vi "Generate Web Service Privilege.vi"(8 "error in (no error)":errorcluster, 10 "Service Name":string, 11 "data.Privilege Mapping":T1(array[cluster])) -> (0 "error out":errorcluster, 3 "resulting string":string)   [LabVIEW 2020, in "Web Service Description.lvlib"]
uses:
  <vilib>/AppBuilder/Engine/WebServiceDescription/Web Service Description.lvlib
  <vilib>/AppBuilder/Engine/WebServiceDescription/XMLGen/XMLGen.lvlib
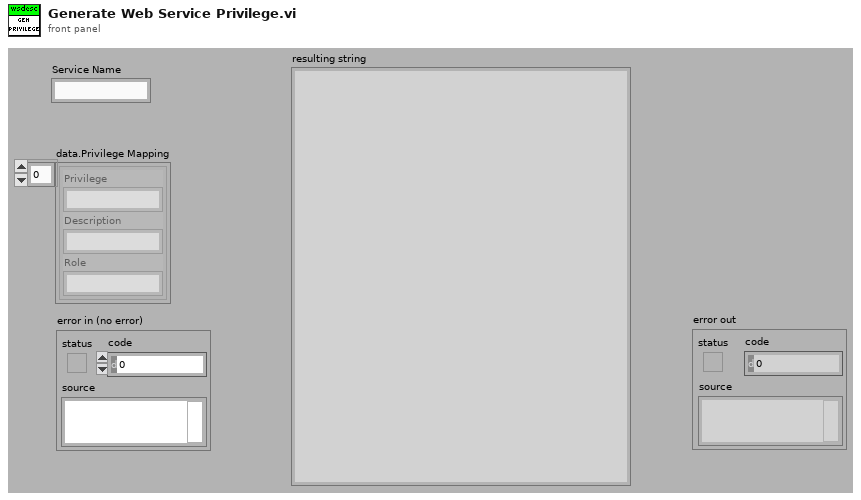
[diagram p1: front panel]
types:
  T1 = cluster{"Privilege":string, "Description":string, "Role":string}[]
  T2 = cluster{"element":string, "XML String Out":string}
  T3 = cluster{"element":string, "XML String Out":string}[]
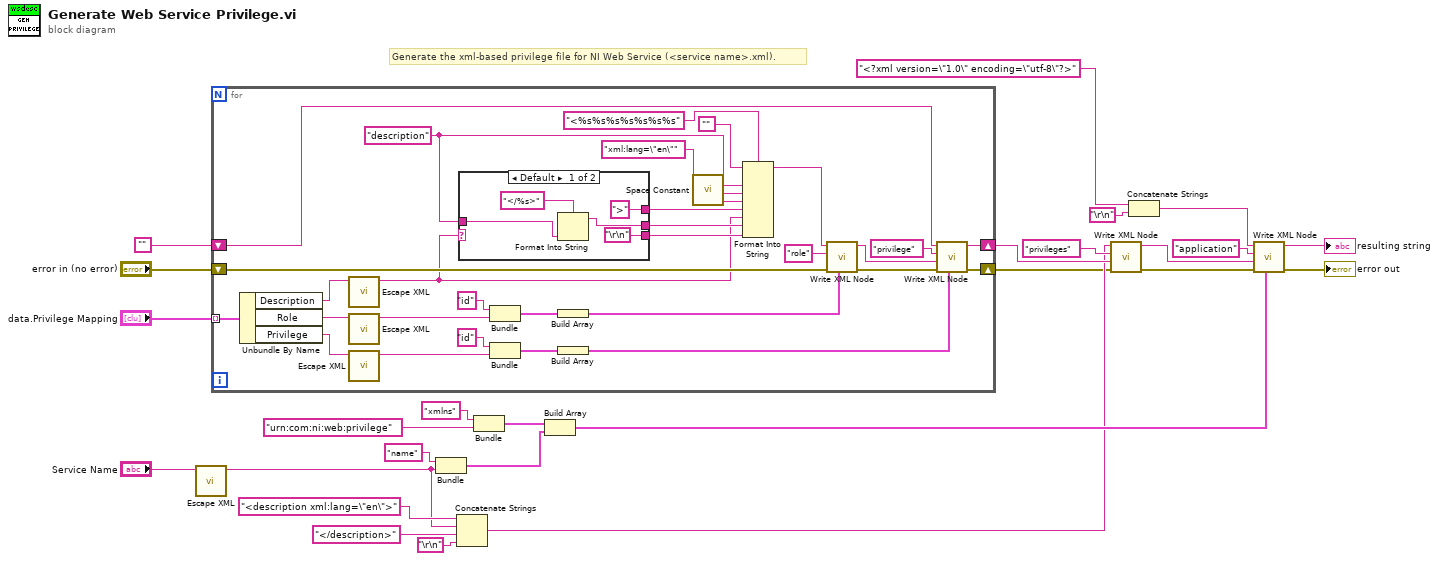
[diagram p0: block diagram]
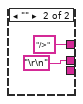
[diagram p2: hidden frame]
diagram:
  # "Generate the xml-based privilege file for NI Web Service (<service name>.xml)."
  n1 = call <vilib>:"Escape XML.vi"("XML String In"="Service Name") -> ("XML String Out"=w1:string)  [unwired: 9 in, 1 out]
  n2 = for {
    tunnel: "data.Privilege Mapping" -> [w56] mode=indexing
    shift-right: [w52] -> w23
    shift-left: "" -> [w48]
    shift-right: [w51] -> w5
    shift-left: "error in (no error)" -> [w42]
    w41 = "description" ("node")
    n3 = Unbundle By Name(w56) -> ("Description"=w32:string, "Role"=w30:string, "Privilege"=w28:string)
    n4 = call <vilib>:"Escape XML.vi"("XML String In"=w32) -> ("XML String Out"=w31:string)  [unwired: 9 in, 1 out]
    n5 = call <vilib>:"Escape XML.vi"("XML String In"=w30) -> ("XML String Out"=w29:string)  [unwired: 9 in, 1 out]
    n6 = call <vilib>:"Escape XML.vi"("XML String In"=w28) -> ("XML String Out"=w27:string)  [unwired: 9 in, 1 out]
    n7 = case shown="Default" w31 {
      tunnel: [w61 "\r\n"] -> w38
      tunnel: w41 -> [w59 _]
      tunnel: [">" "/>"] -> w39
      tunnel: ["\r\n" _] -> w37
      frame Default {
        n8 = Format Into String(format string="</%s>", w59) -> (resulting string=w61:string)  [unwired: 2 in, 1 out]
      }
      frame "" {
      }
    }
    n9 = Bundle("element"="id", "XML String Out"=w29) -> (w45:T2)  [unwired: 1 out]
    n10 = Bundle("id", "XML String Out"=w27) -> (w50:cluster{string, "XML String Out":string})  [unwired: 1 out]
    n11 = Build Array(w45) -> (w46:T3)
    n12 = Build Array(w50) -> (w54:cluster{string, "XML String Out":string}[])
    n13 = call <vilib>:"Space Constant.vi"() -> ("String"=w34:string)
    n14 = Format Into String(format string="<%s%s%s%s%s%s%s", initial string="", w41, w34, "xml:lang=\"en\"", w39, w31, w38, w37) -> (resulting string=w33:string)  [unwired: 1 in, 1 out]
    n15 = call <vilib>:"Write XML Node.vi"("attributes"=w46, "error in (no error)"=w42, "node"="role", "initial string"=w33) -> ("error out"=w43:errorcluster, "resulting string"=w49:string)  [unwired: 1 in, 5 out]
    n16 = call <vilib>:"Write XML Node.vi"("attributes"=w54, "error in (no error)"=w43, "body"=w49, "node"="privilege", "initial string"=w48) -> ("error out"=w51:errorcluster, "resulting string"=w52:string)  [unwired: 5 out]
  }
  n17 = Bundle("name", "XML String Out"=w1) -> (w19:cluster{string, "XML String Out":string})  [unwired: 1 out]
  n18 = Concatenate Strings("<description xml:lang=\"en\">" ("string"), w1, "</description>" ("string"), "\r\n") -> (w9:string)
  n19 = Bundle("xmlns", "urn:com:ni:web:privilege") -> (w14:cluster{string, string})  [unwired: 1 out]
  n20 = Build Array(w14, w19) -> (w18:cluster{string, "XML String Out":string}[])
  n21 = call <vilib>:"Write XML Node.vi"("error in (no error)"=w5, "body"=w23, "node"="privileges", "initial string"=w9) -> ("error out"=w15:errorcluster, "resulting string"=w13:string)  [unwired: 1 in, 5 out]
  n22 = Concatenate Strings("<?xml version=\"1.0\" encoding=\"utf-8\"?>" ("string"), "\r\n") -> (w10:string)
  n23 = call <vilib>:"Write XML Node.vi"("attributes"=w18, "error in (no error)"=w15, "body"=w13, "node"="application", "initial string"=w10) -> ("error out"=→"error out":errorcluster, "resulting string"=→"resulting string":string)  [unwired: 5 out]
